vi "GetStepUIfromConfig.vi"(8 "error in (no error)":errorcluster, 11 "Step Config in":refnum<class "Step Config.lvclass">) -> (0 "error out":errorcluster, 2 "Step UI class name":string, 3 "Step UI out":refnum<class "Step UI.lvclass">)   [LabVIEW 2015, in "StepNode.lvclass"]
uses:
  StepNode.lvclass
  Prototype/classes/Step/UI/Step UI.lvclass
  Prototype/classes/Step/Config/Step Config.lvclass
  Configuration Tool.lvlib
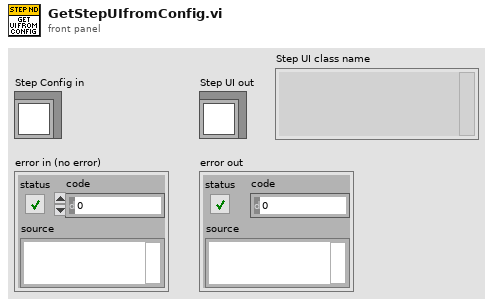
[diagram p1: front panel]
types:
  T1 = typedef "Configuration Tool.lvlib/StepClassLibrary.ctl" = cluster{"Step Types":string[], "Step Config Classes":refnum<class "Step Config.lvclass">[], "Step UI Classes":refnum<class "Step UI.lvclass">[]}
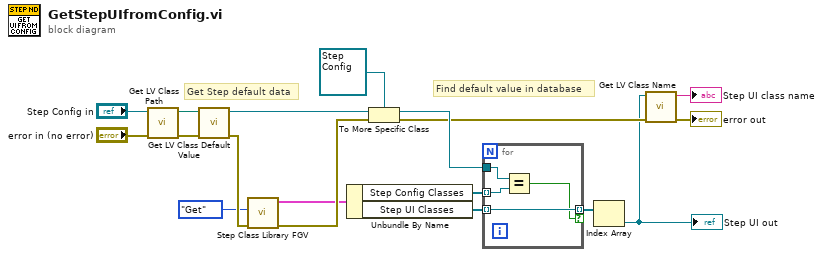
[diagram p0: block diagram]
diagram:
  # "Find default value in database"
  # "Get Step default data"
  n1 = call <vilib>:"Get LV Class Path.vi"("error in (no error)"="error in (no error)", "object"="Step Config in") -> ("error out"=w7:errorcluster, "class path"=w9:path)  [unwired: 8 in]
  n2 = call <vilib>:"Get LV Class Default Value.vi"("error in (no error)"=w7, "class path"=w9) -> ("error out"=w10:errorcluster, "object"=w14:refnum<class>)  [unwired: 8 in]
  n3 = call "Step Class Library FGV.vi"("error in (no error)"=w10, "Action"=enum16{"Set", "Get"}."Get") -> ("error out"=w16:errorcluster, "Step Type Class Library out"=w11:T1)  [unwired: 8 in]
  n4 = Unbundle By Name(w11) -> ("Step Config Classes"=w12:refnum<class "Step Config.lvclass">[], "Step UI Classes"=w13:refnum<class "Step UI.lvclass">[])
  n5 = To More Specific Class(target class=refnum<class "Step Config.lvclass"> refnum ("x"), reference=w14, error in=w16) -> (specific class reference=w15:refnum<class "Step Config.lvclass">, error out=w4:errorcluster)
  n6 = for {
    tunnel: w12 -> [w22] mode=indexing
    tunnel: w13 -> [w20] mode=indexing
    tunnel: w15 -> [w21]
    tunnel: [w20] -> w18 mode=indexing if=w19
    n7 = Equal?(x=w21, y=w22) -> (x = y?=w19:bool)
  }
  n8 = Index Array(array=w18) -> (element=w2:refnum<class "Step UI.lvclass">)  [unwired: 1 in]
  "Step UI out" <- w2
  n9 = call <vilib>:"Get LV Class Name.vi"("error in (no error)"=w4, "object"=w2) -> ("error out"=→"error out":errorcluster, "class name"=→"Step UI class name":string)  [unwired: 8 in]
